vi "Temperature Multiplot.vi"() -> ()   [LabVIEW 2014]
doc: "This VI is the solution to an exercise in the LabVIEW Core I course.\n\nIt is used to demonstrate While loops and waveform charts. This VI simulates a temperature reading once every 500 ms and plots the data in a strip chart."
panel:
  out "Temperature History":cluster{dbl, "Temperature":dbl}(graph)
  in  "Power":bool=TRUE
  # "ON\n\nOFF"
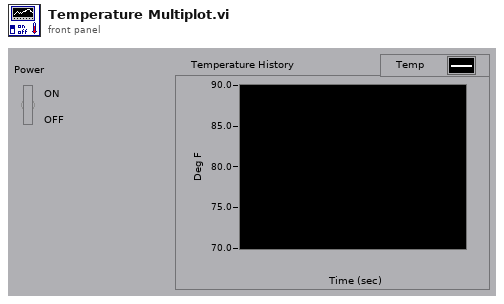
[diagram p1: front panel]
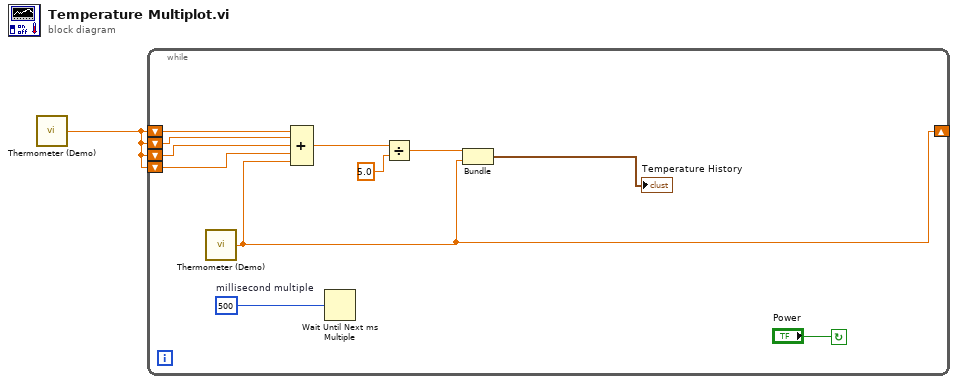
[diagram p0: block diagram]
diagram:
  n1 = call "Thermometer (Demo).vi"() -> ("Temperature"=w1:dbl)  [unwired: 1 in]
  n2 = while {
    shift-right: [w3] -> _
    shift-left: w1 -> [w10]
    shift-left: w1 -> [w9]
    shift-left: w1 -> [w7]
    shift-left: w1 -> [w8]
    stop <- "Power" continue-if-true
    w11 = u32 500  # millisecond multiple
    n3 = call "Thermometer (Demo).vi"() -> ("Temperature"=w3:dbl)  [unwired: 1 in]
    n4 = Compound Arithmetic op=ADD(w10, w9, w8, w7, w3) -> (w2:dbl)
    n5 = Wait Until Next ms Multiple(millisecond multiple=w11) -> ()  [unwired: 1 out]
    n6 = Divide(x=w2, y=5.0 ("x/y")) -> (x/y=w5:dbl)
    n7 = Bundle(w5, "Temperature"=w3) -> (→"Temperature History":cluster{dbl, "Temperature":dbl})  [unwired: 1 in]
  }
